vi "PIDAutoTune_Convert_Academic_To_NonInteracting.vi"(9 "Kn":dbl, 11 "PID gains NI Academic":T2) -> (3 "PID Gains Non Interacting":T1)   [LabVIEW 2019, in "Trajectory_Library.lvlib"]
uses:
  Trajectory_Library.lvlib
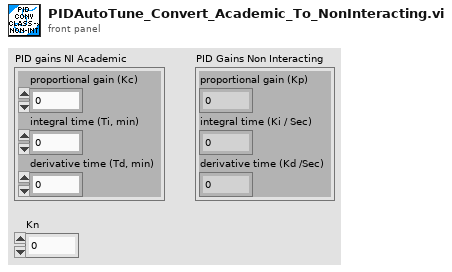
[diagram p1: front panel]
types:
  T1 = cluster{"proportional gain (Kp)":dbl, "integral time (Ki / Sec)":dbl, "derivative time (Kd /Sec)":dbl}
  T2 = cluster{"proportional gain (Kc)":dbl, "integral time (Ti, min)":dbl, "derivative time (Td, min)":dbl}
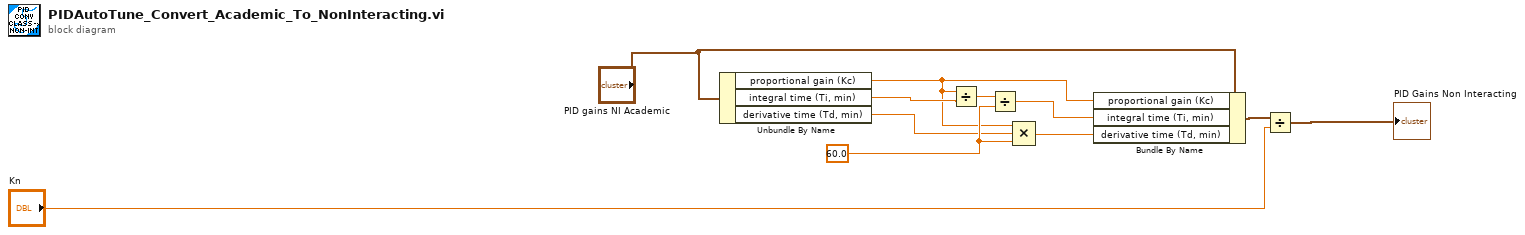
[diagram p0: block diagram]
diagram:
  w5 = 60.0 ("y")
  n1 = Unbundle By Name("PID gains NI Academic") -> ("proportional gain (Kc)"=w4:dbl, "integral time (Ti, min)"=w8:dbl, "derivative time (Td, min)"=w3:dbl)
  n2 = Divide(x=w4, y=w8) -> (x/y=w7:dbl)
  n3 = Divide(x=w7, y=w5) -> (x/y=w6:dbl)
  n4 = Compound Arithmetic op=MULTIPLY(w4, w3, w5) -> (w2:dbl)
  n5 = Bundle By Name(cluster="PID gains NI Academic", "proportional gain (Kc)"=w4, "integral time (Ti, min)"=w6, "derivative time (Td, min)"=w2) -> (w1:T2)
  n6 = Divide(x=w1, y="Kn") -> (x/y=→"PID Gains Non Interacting":T2)
